vi "Stop.vi"(8 "error in (no error)":errorcluster, 11 "Execution in":refnum<data-value>) -> (0 "error out":errorcluster, 3 "Execution out":refnum<data-value>)   [LabVIEW 2015, in "Execution.lvclass"]
uses:
  Execution.lvclass
  EXECUTION_CTRL_MSG.ctl
  EXECUTION_UI_MSG.ctl
  Send Control Message.vi
  Send UI Message.vi
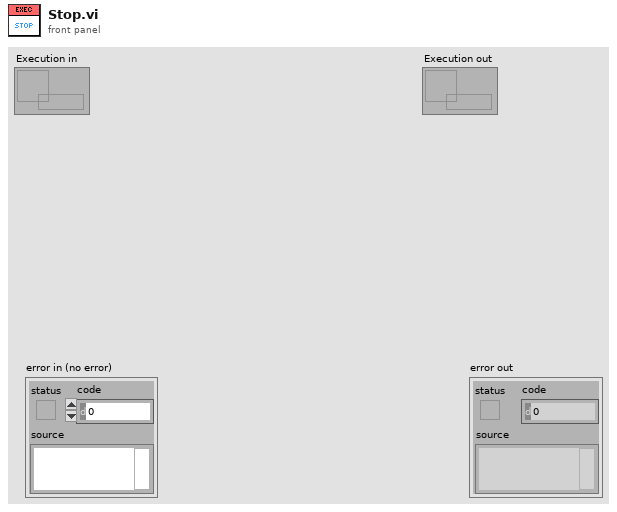
[diagram p1: front panel]
types:
  T1 = typedef "Execution.lvclass/EXECUTION_UI_MSG.ctl" = enum16{"EXECUTION_STATUS", "INIT_UI", "DUT_UPDATE", "BOTTOM_PANEL_UPDATE", "TOP_PANEL_UPDATE", "STEP_START", "STEP_END", "DISPLAY_RESULT", "APPLICATION_END"}
  T2 = typedef "Execution.lvclass/EXECUTION_CTRL_MSG.ctl" = enum16{"EXECUTION_START", "EXECUTION_END", "EXECUTION_LOOP", "APPLICATION_STOP"}
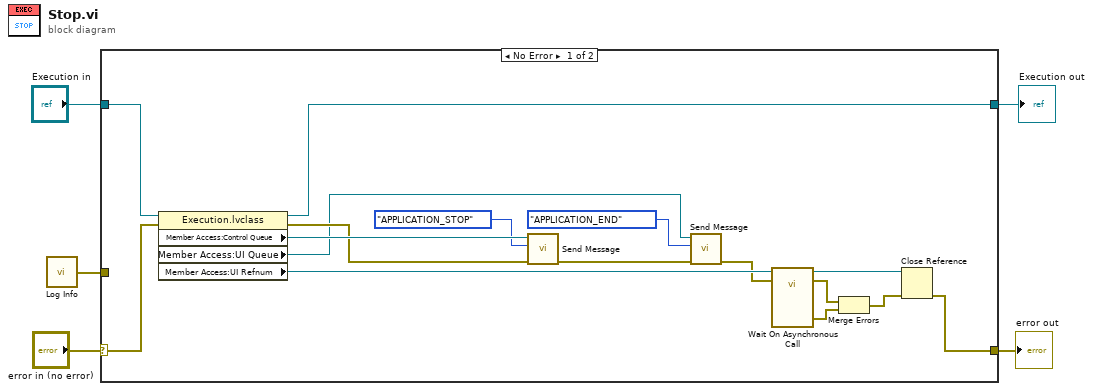
[diagram p0: block diagram]
diagram:
  n1 = call "Log Info.vi"() -> ("error out"=w1:errorcluster)  [unwired: 5 in]
  n2 = case shown="No Error" "error in (no error)" {
    selector: "error in (no error)" -> [w15 w23]
    tunnel: [w14 w23] -> w4
    tunnel: [w16 w22] -> w2
    tunnel: "Execution in" -> [w21 w22]
    tunnel: w1 -> [_ _]
    frame No Error {
      n3 = property class="Execution.lvclass"(reference=w21, error in=w15) -> (reference out=w16:refnum<data-value>, error out=w10:errorcluster, "Member Access:Control Queue"=w12:refnum<queue>, "Member Access:UI Queue"=w7:refnum<queue>, "Member Access:UI Refnum"=w13:refnum<vi>)
      n4 = call-poly "Send Message.vi"("error in (no error)"=w10, "Msg"=EXECUTION_CTRL_MSG."APPLICATION_STOP", "Control Queue"=w12) -> ("error out"=w9:errorcluster)  [unwired: 8 in]
      n5 = call-poly "Send Message.vi"("error in (no error)"=w9, "Msg"=EXECUTION_UI_MSG."APPLICATION_END", "UI Queue"=w7) -> ("error out"=w8:errorcluster)  [unwired: 8 in]
      n6 = call-by-ref "Wait On Asynchronous Call"(reference=w13, error in=w8) -> (reference out=w17:refnum<vi>, error out=w18:errorcluster, 0:"error out"=w19:errorcluster)  [unwired: 10 in, 1 out]
      n7 = Merge Errors(w18, w19) -> (w20:errorcluster)
      n8 = Close Reference(reference=w17, error in (no error)=w20) -> (error out=w14:errorcluster)
    }
    frame Error {
    }
  }
  "error out" <- w4
  "Execution out" <- w2
